vi "Fix Warning.vi"(8 "Error In":errorcluster, 9 "Warning Index":i32, 10 "Warnings":T1[](array[typedef]), 11 "Install LV Data in":T2={"SSH Session"=refnum, "Status Log"="", "Detailed Log"="", "Credentials"={"Hostname or IP"="192.168.7.2", "Username"="root", "Password"=""}, "Target Info"={"OS Version"="", "CPU"="", "Systemd Version"="", "Internet Access"=FALSE, "Device Type"="", "LV Installed Ver"="", "LV Available Ver"="", "LV Upgrade Available"=FALSE, "Hostname"="", "NIC Info"=[]}, "Reboot Required?"=FALSE}) -> (0 "Error Out":errorcluster, 1 "Visible Index":i32, 2 "Warnings":T1[](array[typedef]), 3 "Install LV Data out":T2={"SSH Session"=refnum, "Status Log"="", "Detailed Log"="", "Credentials"={"Hostname or IP"="192.168.7.2", "Username"="root", "Password"=""}, "Target Info"={"OS Version"="", "CPU"="", "Systemd Version"="", "Internet Access"=FALSE, "Device Type"="", "LV Installed Ver"="", "LV Available Ver"="", "LV Upgrade Available"=FALSE, "Hostname"="", "NIC Info"=[]}, "Reboot Required?"=FALSE})   [LabVIEW 2014, in "LMH-LINX.lvlib"]
uses:
  <vilib>/MakerHub/LINX/LMH-LINX.lvlib
  <vilib>/MakerHub/LINX/Private/Utilties/Target Management/Target Compatibility Warnings.ctl
  <vilib>/MakerHub/LINX/Private/Utilties/Target Management/Install LV Data.ctl
  C:/Program Files (x86)/National Instruments/LabVIEW 2014/vi.lib/MakerHub/LINX/Resources/Renci.SshNet.dll
  Resources/Renci.SshNet.dll
  <vilib>/MakerHub/LINX/Private/Utilties/Target Management/Target Info.ctl
  <vilib>/MakerHub/LINX/Private/Utilties/Target Management/NIC Info.ctl
  <vilib>/MakerHub/LINX/Private/Utilties/Target Management/NIC Mode.ctl
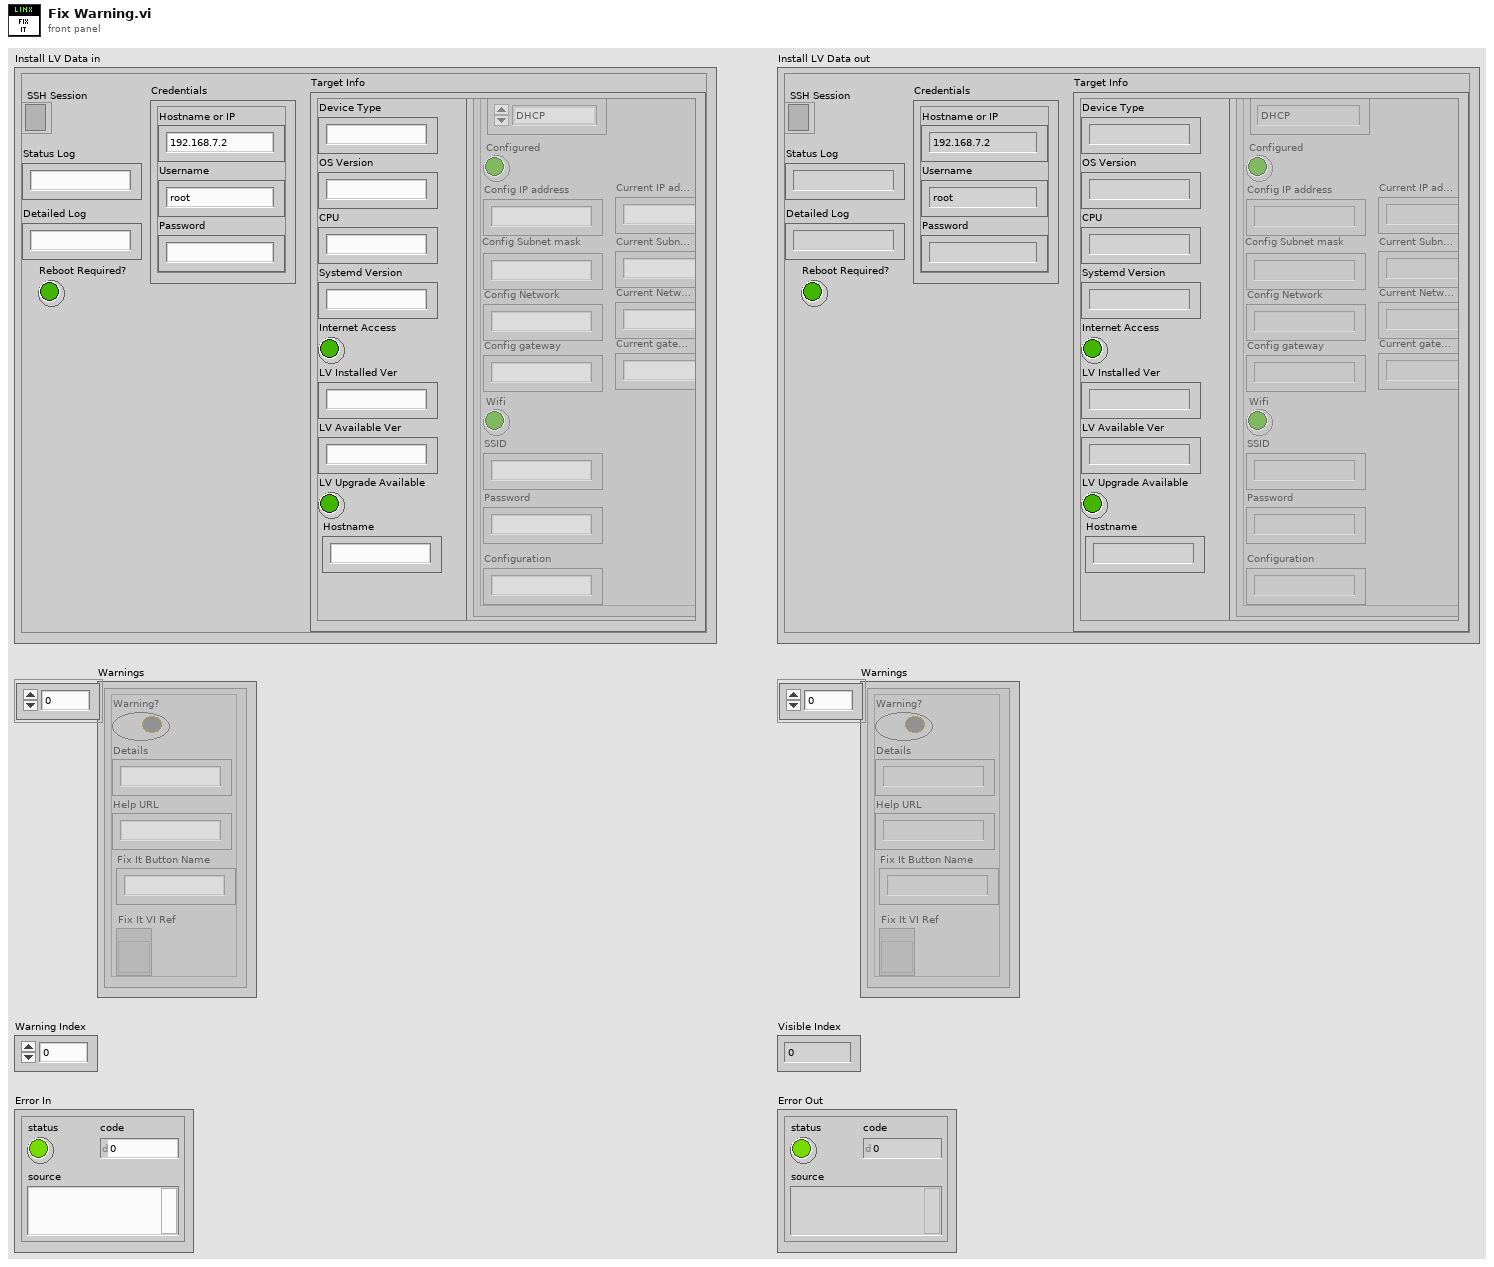
[diagram p1: front panel]
types:
  T1 = typedef "LMH-LINX.lvlib/Target Compatibility Warnings.ctl" = cluster{"Warning?":bool, "Details":string, "Help URL":string, "Fix It Button Name":string, "Fix It VI Ref":refnum<vi>}
  T2 = typedef "LMH-LINX.lvlib/Install LV Data.ctl" = cluster{"SSH Session":refnum<k24>, "Status Log":string, "Detailed Log":string, "Credentials":cluster{"Hostname or IP":string, "Username":string, "Password":string}, "Target Info":T3, "Reboot Required?":bool}
  T3 = typedef "LMH-LINX.lvlib/Target Info.ctl" = cluster{"OS Version":string, "CPU":string, "Systemd Version":string, "Internet Access":bool, "Device Type":string, "LV Installed Ver":string, "LV Available Ver":string, "LV Upgrade Available":bool, "Hostname":string, "NIC Info":T4[]}
  T4 = typedef "LMH-LINX.lvlib/NIC Info.ctl" = cluster{"Name":string, "NIC Mode":T5, "Configured":bool, "Config IP address":string, "Config Subnet mask":string, "Config Network":string, "Config gateway":string, "Wifi":bool, "SSID":string, "Password":string, "Configuration":string, "Current IP address":string, "Current Subnet mask":string, "Current gateway":string, "Current Network":string}
  T5 = typedef "LMH-LINX.lvlib/NIC Mode.ctl" = enum16{"DHCP", "Static", "Loopback"}
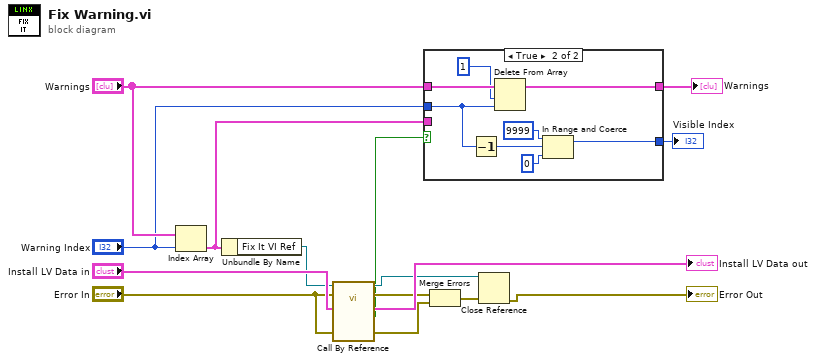
[diagram p0: block diagram]
diagram:
  n1 = Index Array(array="Warnings", index="Warning Index") -> (element=w4:T1)
  n2 = Unbundle By Name(w4) -> ("Fix It VI Ref"=w7:refnum<vi>)
  n3 = call-by-ref "?"(reference=w7, error in="Error In", "Error In"="Error In", "Install LV Data"="Install LV Data in") -> (reference out=w12:refnum<vi>, error out=w9:errorcluster, "Error Out"=w10:errorcluster, "Fixed?"=w3:bool, "Install LV Data"=→"Install LV Data out":T2)  [unwired: 7 in]
  n4 = case shown="True" w3 {
    tunnel: "Warnings" -> [w17 w25]
    tunnel: "Warning Index" -> [w16 w22]
    tunnel: w4 -> [_ _]
    tunnel: [w17 w23] -> w2
    tunnel: [w16 w18] -> w1
    frame False {
    }
    frame True {
      n5 = Decrement(x=w22) -> (x-1=w21:i32)
      n6 = Delete From Array(array=w25, length=1, index=w22) -> (array with subset deleted=w23:T1[])  [unwired: 1 out]
      n7 = In Range and Coerce(upper limit=9999, x=w21, lower limit=0) -> (coerced(x)=w18:i32)  [unwired: 1 out]
    }
  }
  "Warnings" <- w2
  "Visible Index" <- w1
  n8 = Merge Errors(w9, w10) -> (w11:errorcluster)
  n9 = Close Reference(reference=w12, error in (no error)=w11) -> (error out=→"Error Out":errorcluster)
